vi "FPGAref.vi"(4 "error in":errorcluster, 6 "Enum":enum16{"Set", "Get"}(ring)=enum."Get", 7 "FPGA VI Reference Out":refnum<k20>) -> (0 "error out":errorcluster, 3 "FPGA VI Reference Out 2":refnum<k20>)   [LabVIEW 2019]
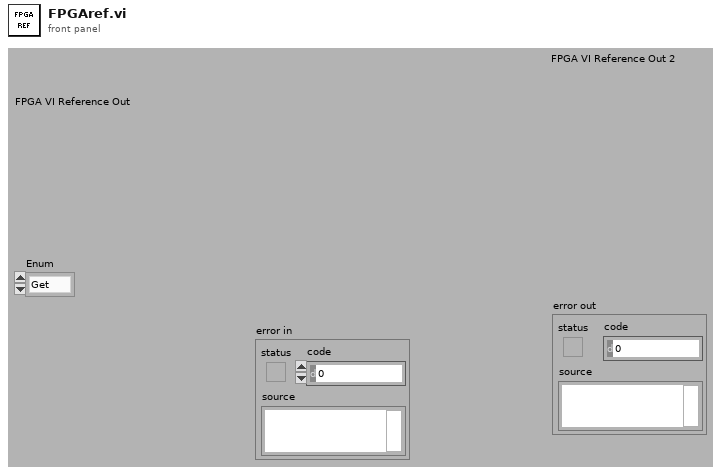
[diagram p1: front panel]
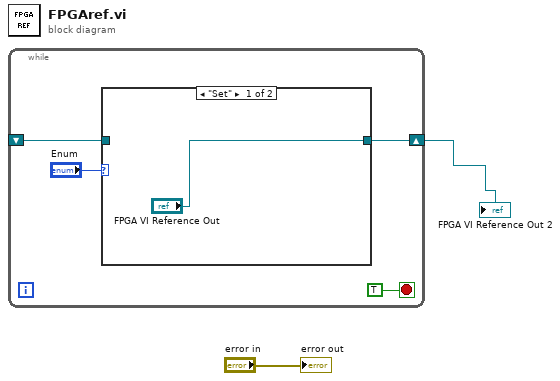
[diagram p0: block diagram]
diagram:
  n1 = while {
    shift-right: [w4] -> w1
    shift-left: _ -> [w3]
    stop <- TRUE stop-if-true
    n2 = case shown="\"Set\"" "Enum" {
      tunnel: ["FPGA VI Reference Out" w8] -> w4
      tunnel: w3 -> [_ w8]
      frame "Set" {
      }
      frame "Get", Default {
      }
    }
  }
  "FPGA VI Reference Out 2" <- w1
  "error out" <- "error in"
